vi "P4CMD Execute Command.vi"(5 "optional operation parameters":string, 6 "operation message":string, 7 "p4 operation":T2, 8 "error in (no error)":errorcluster, 9 "input string":string, 10 "files":path[](array[path]), 11 "source control reference in":T1) -> (0 "error out":errorcluster, 2 "command information":string, 3 "source control reference out":T1)   [LabVIEW 2020, in "NI_SCC_P4CMD.lvlib"]
uses:
  <vilib>/SourceControl/Providers/P4CMD/NI_SCC_P4CMD.lvlib
  <vilib>/SourceControl/Providers/P4CMD/P4CMD Operations.ctl
  <vilib>/SourceControl/sccapi/SCCAPI Refnum.ctl
  <vilib>/SourceControl/Providers/P4CMD/P4CMD Mgr Functions.ctl
  <vilib>/SourceControl/sccapi/NI_SCC.lvlib
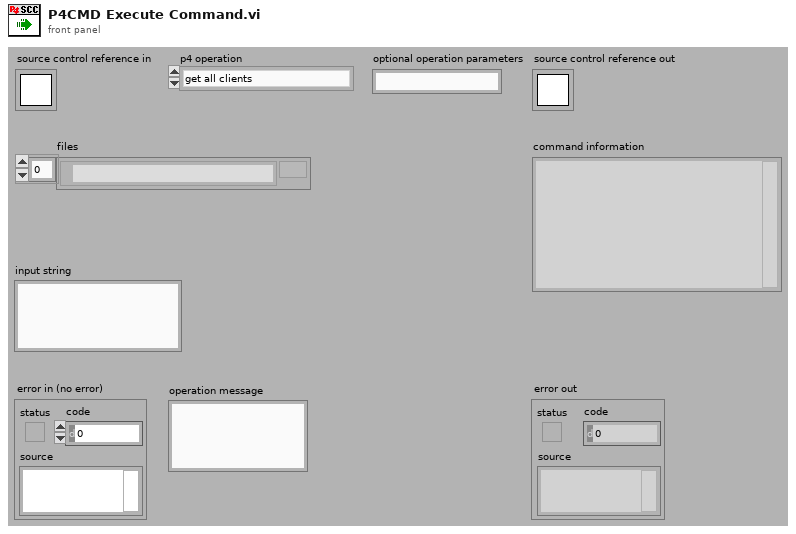
[diagram p1: front panel]
types:
  T1 = typedef "NI_SCC.lvlib/SCCAPI Refnum.ctl" = refnum<k1>
  T2 = typedef "NI_SCC_P4CMD.lvlib/P4CMD Operations.ctl" = enum16{"get all clients", "get all users", "describe changelist", "sync from depot", "open for edit", "submit to depot", "revert", "add to depot", "remove from depot", "print files revisions", "compare client file", "print depot file contents", "list opened files", "get file info", "lock files", "edit changelist spec", "info", "set variables"}
  T3 = typedef "NI_SCC_P4CMD.lvlib/P4CMD Mgr Functions.ctl" = enum16{"Init", "Open", "Set Config Opts", "Initialized?", "IsRefValid?", "Get Config Opts", "Get Global Commands", "Close", "Uninit"}
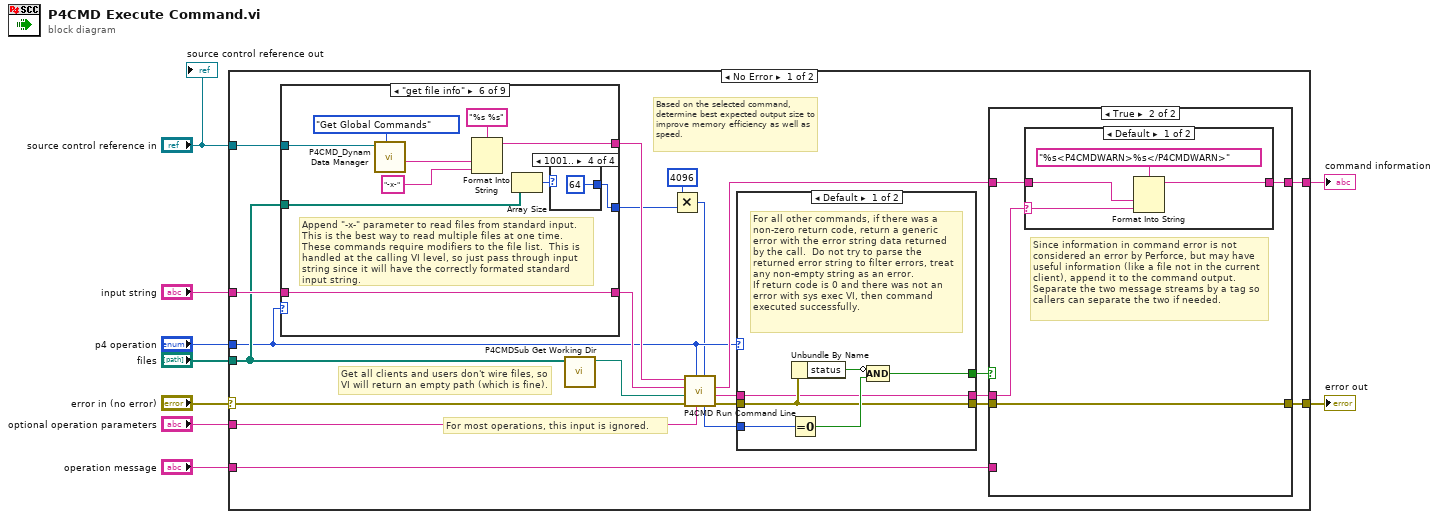
[diagram p0: block diagram]
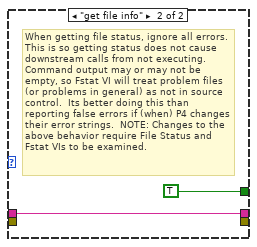
[diagram p2: hidden frame]
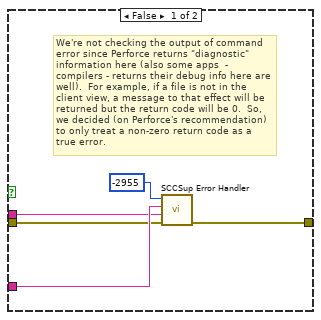
[diagram p3: hidden frame]
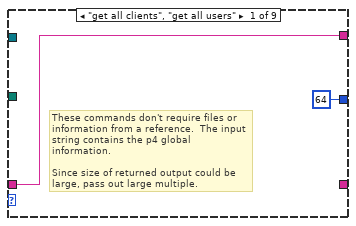
[diagram p5: hidden frame]
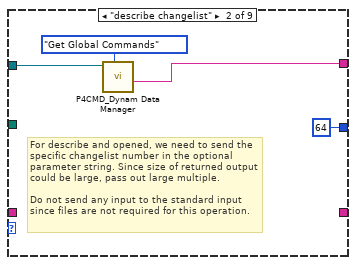
[diagram p6: hidden frame]
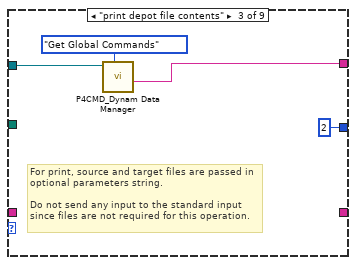
[diagram p7: hidden frame]
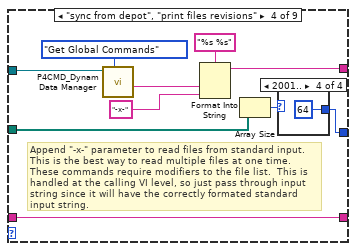
[diagram p8: hidden frame]
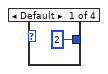
[diagram p9: hidden frame]
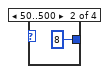
[diagram p10: hidden frame]
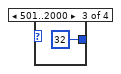
[diagram p11: hidden frame]
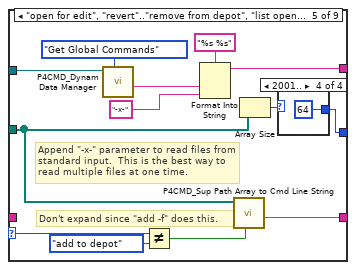
[diagram p12: hidden frame]
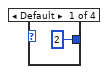
[diagram p13: hidden frame]
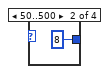
[diagram p14: hidden frame]
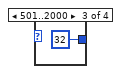
[diagram p15: hidden frame]
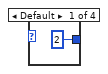
[diagram p16: hidden frame]
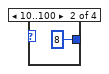
[diagram p17: hidden frame]
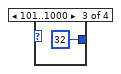
[diagram p18: hidden frame]
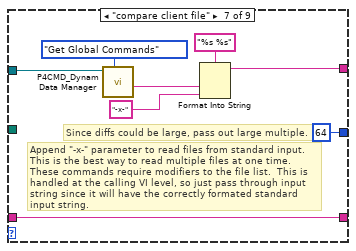
[diagram p19: hidden frame]
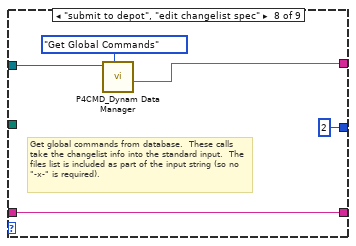
[diagram p20: hidden frame]
diagram:
  n1 = case shown="No Error" "error in (no error)" {
    selector: "error in (no error)" -> [w24 w123]
    tunnel: "source control reference in" -> [w31 _]
    tunnel: "input string" -> [w30 _]
    tunnel: "files" -> [w23 _]
    tunnel: [w17 _] -> w6
    tunnel: [w26 w123] -> w5
    tunnel: "operation message" -> [w21 _]
    tunnel: "p4 operation" -> [w16 _]
    tunnel: "optional operation parameters" -> [w20 _]
    frame No Error {
      # "Based on the selected command, determine best expected output size to improve memory efficiency as well as speed."
      # "For most operations, this input is ignored."
      # "Get all clients and users don't wire files, so VI will return an empty path (which is fine)."
      n2 = case shown="\"get file info\"" w16 {
        selector: w16 -> [_ _ _ _ w83 _ _ _ _]
        tunnel: w31 -> [_ w58 w62 w69 w86 w100 w112 w119 _]
        tunnel: w30 -> [w55 _ _ w67 _ w98 w110 w121 _]
        tunnel: w23 -> [_ _ _ w65 w78 w96 _ _ _]
        tunnel: [w55 w57 w61 w68 w85 w99 w111 w118 _] -> w29
        tunnel: [_ _ _ w67 w84 w98 w110 w121 _] -> w28
        tunnel: [u32 64 ("y") u32 64 ("y") u32 2 ("y") w64 w79 w95 u32 64 ("y") u32 2 ("y") u32 2 ("y")] -> w12
        frame "get all clients", "get all users" {
          # "These commands don't require files or information from a reference.  The input string contains the p4 global information.\n\nSince size of returned output could be large, pass out large multiple."
        }
        frame "describe changelist" {
          # "For describe and opened, we need to send the specific changelist number in the optional parameter string. Since size of returned output could be large, pass out large multiple.\n\nDo not send any input to the standard input since files are not required for this operation."
          n3 = call <vilib>:"P4CMD_Dynam Data Manager.vi"("function"=P4CMD_Mgr_Functions."Get Global Commands", "source control reference in"=w58) -> ("global commands"=w57:string)  [unwired: 4 in, 5 out]
        }
        frame "print depot file contents" {
          # "For print, source and target files are passed in optional parameters string.\n\nDo not send any input to the standard input since files are not required for this operation."
          n4 = call <vilib>:"P4CMD_Dynam Data Manager.vi"("function"=P4CMD_Mgr_Functions."Get Global Commands", "source control reference in"=w62) -> ("global commands"=w61:string)  [unwired: 4 in, 5 out]
        }
        frame "sync from depot", "print files revisions" {
          # "Append \"-x-\" parameter to read files from standard input.  This is the best way to read multiple files at one time.  These commands require modifiers to the file list.  This is handled at the calling VI level, so just pass through input string since it will have the correctly formated standard input string."
          n5 = call <vilib>:"P4CMD_Dynam Data Manager.vi"("function"=P4CMD_Mgr_Functions."Get Global Commands", "source control reference in"=w69) -> ("global commands"=w70:string)  [unwired: 4 in, 5 out]
          n6 = Format Into String(format string="%s %s", w70, "-x-" ("format string")) -> (resulting string=w68:string)  [unwired: 2 in, 1 out]
          n7 = Array Size(array=w65) -> (size(s)=w66:i32)
          n8 = case shown="2001.." w66 {
            tunnel: [u32 2 ("expected output size") u32 8 ("expected output size") u32 32 ("expected output size") u32 64 ("expected output size")] -> w64
            frame Default {
            }
            frame 50..500 {
            }
            frame 501..2000 {
            }
            frame 2001.. {
            }
          }
        }
        frame "open for edit", "revert".."remove from depot", "list opened files", "lock files" {
          # "Don't expand since \"add -f\" does this."
          # "Append \"-x-\" parameter to read files from standard input.  This is the best way to read multiple files at one time."
          n9 = call <vilib>:"P4CMD_Dynam Data Manager.vi"("function"=P4CMD_Mgr_Functions."Get Global Commands", "source control reference in"=w86) -> ("global commands"=w87:string)  [unwired: 4 in, 5 out]
          n10 = Not Equal?(x=w83, y=P4CMD_Operations."add to depot") -> (x != y?=w82:bool)
          n11 = Format Into String(format string="%s %s", w87, "-x-" ("format string")) -> (resulting string=w85:string)  [unwired: 2 in, 1 out]
          n12 = call <vilib>:"P4CMD_Sup Path Array to Cmd Line String.vi"("expand wildcards? (T)"=w82, "files"=w78) -> ("string output"=w84:string)  [unwired: 1 in, 8 out]
          n13 = Array Size(array=w78) -> (size(s)=w80:i32)
          n14 = case shown="2001.." w80 {
            tunnel: [u32 2 ("expected output size") u32 8 ("expected output size") u32 32 ("expected output size") u32 64 ("expected output size")] -> w79
            frame Default {
            }
            frame 50..500 {
            }
            frame 501..2000 {
            }
            frame 2001.. {
            }
          }
        }
        frame "get file info" {
          # "Append \"-x-\" parameter to read files from standard input.  This is the best way to read multiple files at one time.  These commands require modifiers to the file list.  This is handled at the calling VI level, so just pass through input string since it will have the correctly formated standard input string."
          n15 = call <vilib>:"P4CMD_Dynam Data Manager.vi"("function"=P4CMD_Mgr_Functions."Get Global Commands", "source control reference in"=w100) -> ("global commands"=w101:string)  [unwired: 4 in, 5 out]
          n16 = Format Into String(format string="%s %s", w101, "-x-" ("format string")) -> (resulting string=w99:string)  [unwired: 2 in, 1 out]
          n17 = Array Size(array=w96) -> (size(s)=w97:i32)
          n18 = case shown="1001.." w97 {
            tunnel: [u32 2 ("expected output size") u32 8 ("expected output size") u32 32 ("expected output size") u32 64 ("expected output size")] -> w95
            frame Default {
            }
            frame 10..100 {
            }
            frame 101..1000 {
            }
            frame 1001.. {
            }
          }
        }
        frame "compare client file" {
          # "Since diffs could be large, pass out large multiple."
          # "Append \"-x-\" parameter to read files from standard input.  This is the best way to read multiple files at one time.  These commands require modifiers to the file list.  This is handled at the calling VI level, so just pass through input string since it will have the correctly formated standard input string."
          n19 = call <vilib>:"P4CMD_Dynam Data Manager.vi"("function"=P4CMD_Mgr_Functions."Get Global Commands", "source control reference in"=w112) -> ("global commands"=w113:string)  [unwired: 4 in, 5 out]
          n20 = Format Into String(format string="%s %s", w113, "-x-" ("format string")) -> (resulting string=w111:string)  [unwired: 2 in, 1 out]
        }
        frame "submit to depot", "edit changelist spec" {
          # "Get global commands from database.  These calls take the changelist info into the standard input.  The files list is included as part of the input string (so no \"-x-\" is required)."
          n21 = call <vilib>:"P4CMD_Dynam Data Manager.vi"("function"=P4CMD_Mgr_Functions."Get Global Commands", "source control reference in"=w119) -> ("global commands"=w118:string)  [unwired: 4 in, 5 out]
        }
        frame "info", "set variables" {
          # "No additional information is needed for these commands."
        }
      }
      n22 = call <vilib>:"P4CMDSub Get Working Dir.vi"("files"=w23) -> ("working directory"=w22:path)  [unwired: 10 out]
      n23 = Multiply(x=u32 4096 ("expected output size"), y=w12) -> (x*y=w10:u32)
      n24 = call <vilib>:"P4CMD Run Command Line.vi"("expected output size"=w10, "optional operation parameters"=w20, "p4 operation"=w16, "error in (no error)"=w24, "working dir"=w22, "standard input"=w28, "p4 global"=w29) -> ("error out"=w19:errorcluster, "command error output"=w15:string, "command output"=w18:string, "return code"=w27:i32)  [unwired: 1 out]
      n25 = case shown="Default" w16 {
        tunnel: w27 -> [w37 _]
        tunnel: [w36 TRUE] -> w25
        tunnel: w19 -> [w33 _]
        tunnel: w15 -> [w32 w39]
        tunnel: [w32 w39] -> w14
        tunnel: [w33 _] -> w13
        frame Default {
          # "For all other commands, if there was a non-zero return code, return a generic error with the error string data returned by the call.  Do not try to parse the returned error string to filter errors, treat any non-empty string as an error. \nIf return code is 0 and there was not an error with sys exec VI, then command executed successfully."
          n26 = Equal To 0?(x=w37) -> (x = 0?=w34:bool)
          n27 = Unbundle By Name(w33) -> ("status"=w35:bool)
          n28 = Compound Arithmetic op=AND(invert w35, w34) -> (w36:bool)
        }
        frame "get file info" {
          # "When getting file status, ignore all errors.  This is so getting status does not cause downstream calls from not executing.  Command output may or may not be empty, so Fstat VI will treat problem files (or problems in general) as not in source control.  Its better doing this than reporting false errors if (when) P4 changes their error strings.  NOTE: Changes to the above behavior require File Status and Fstat VIs to be examined."
        }
      }
      n29 = case shown="True" w25 {
        tunnel: w13 -> [w42 w48]
        tunnel: [w44 w48] -> w26
        tunnel: w14 -> [w41 w47]
        tunnel: w21 -> [w43 _]
        tunnel: w18 -> [_ w46]
        tunnel: [_ w45] -> w17
        frame False {
          # "We're not checking the output of command error since Perforce returns \"diagnostic\" information here (also some apps  - compilers - returns their debug info here are well).  For example, if a file is not in the client view, a message to that effect will be returned but the return code will be 0.  So, we decided (on Perforce's recommendation) to only treat a non-zero return code as a true error."
          n30 = call <vilib>:"SCCSup Error Handler.vi"("error in (no error)"=w42, "additional message"=w41, "operation message"=w43, "scc error code"=-2955 ("error code")) -> ("error out"=w44:errorcluster)  [unwired: 7 out]
        }
        frame True {
          # "Since information in command error is not considered an error by Perforce, but may have useful information (like a file not in the current client), append it to the command output.   Separate the two message streams by a tag so callers can separate the two if needed."
          n31 = case shown="Default" w47 {
            selector: w47 -> [w50 _]
            tunnel: w46 -> [w51 w53]
            tunnel: [w49 w53] -> w45
            frame Default {
              n32 = Format Into String(format string="%s<P4CMDWARN>%s</P4CMDWARN>", w51, w50) -> (resulting string=w49:string)  [unwired: 2 in, 1 out]
            }
            frame "" {
            }
          }
        }
      }
    }
    frame Error {
    }
  }
  "error out" <- w5
  "command information" <- w6
  "source control reference out" <- "source control reference in"
